vi "BehaviorLineColor.vi"(11 "Select Your Behavior":T2(ring)) -> (2 "line style":T1, 3 "color(":u32)   [LabVIEW 2010]
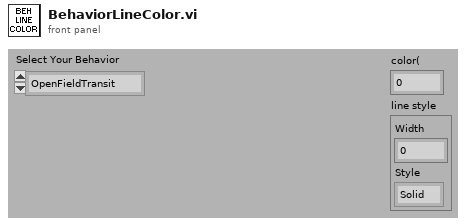
[diagram p1: front panel]
types:
  T1 = cluster{"Width":u16, "Style":enum32{"Solid", "Dash", "Dot", "DashDot", "DashDotDot"}}
  T2 = enum16{"OpenFieldTransit", "WallFollow", "LaneFollow", "ManualMode"}
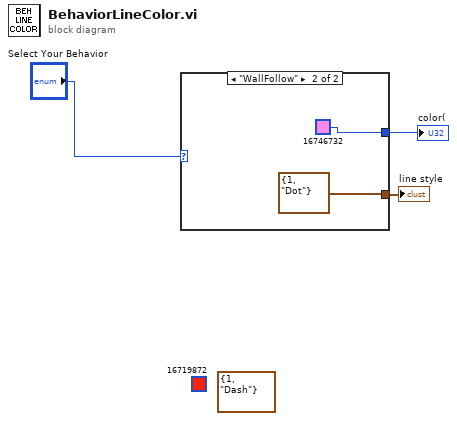
[diagram p0: block diagram]
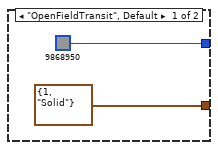
[diagram p2: hidden frame]
diagram:
  (unwired) T1 {"Width"=1, "Style"=enum."Dash"} ("pen")
  (unwired) u32 16719872 ("color(black)")
  n1 = case shown="\"WallFollow\"" "Select Your Behavior" {
    tunnel: [u32 9868950 ("color(black)") u32 16746732 ("color(black)")] -> w2
    tunnel: [T1 {"Width"=1, "Style"=enum."Solid"} ("pen") T1 {"Width"=1, "Style"=enum."Dot"} ("pen")] -> w1
    frame "OpenFieldTransit", Default {
    }
    frame "WallFollow" {
    }
  }
  "color(" <- w2
  "line style" <- w1
